vi "GlobalVar_LED.vi"() -> ()   [LabVIEW 2016]
uses:
  TypeDefs/GearCollectState_Type.ctl
  TypeDefs/GearPlaceState_Type.ctl
  TypeDefs/TurretAimState_Type.ctl
  TypeDefs/AutoMode_Type.ctl
panel:
  in  "AutoMode":T1
  out "UltraPosition":u8
  out "YoYoPosition":u8
  out "Climbing":bool
  out "Shooting":bool
  out "TurretAimed":bool
  out "Turret_State":T2=enum."SearchLeft"
  in  "Win":bool
  out "GearPlace_State":T3
  out "GearCatch_State":T4
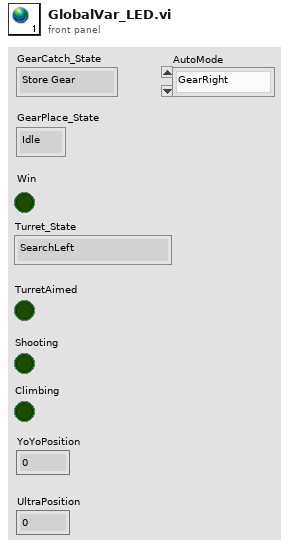
[diagram p1: front panel]
types:
  T1 = typedef "AutoMode_Type.ctl" = enum16{"GearRight", "GearMiddle", "GearLeft"}
  T2 = typedef "TurretAimState_Type.ctl" = enum16{"Idle", "SearchLeft", "SearchRight", "FindNewTarget", "TargetAcquired"}
  T3 = typedef "GearPlaceState_Type.ctl" = enum16{"Idle", "Wait for Peg", "Allign To Lift", "Arm Gear", "Place Gear", "Return to Ready", "Disarm Gear"}
  T4 = typedef "GearCollectState_Type.ctl" = enum16{"Store Gear", "Wait For Gear", "Idle"}
diagram:
